vi "AddSystemIDtoCaliFile.vi"() -> ()   [LabVIEW 2020]
panel:
  out "error out":errorcluster
  in  "SYstemID":string(combo)="UCDMC"
  in  "error in (no error)":errorcluster
  out "selected path":path
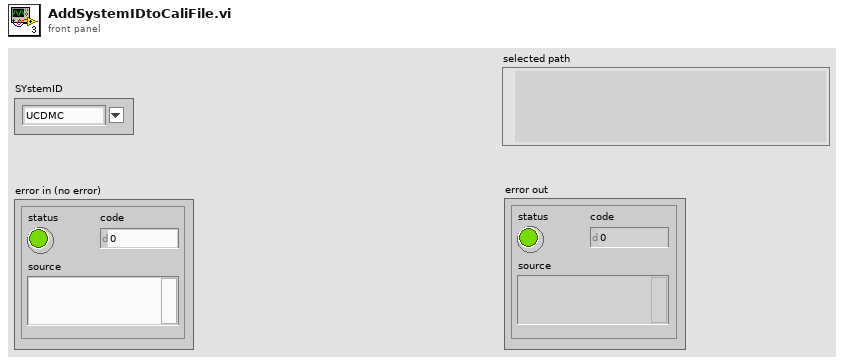
[diagram p1: front panel]
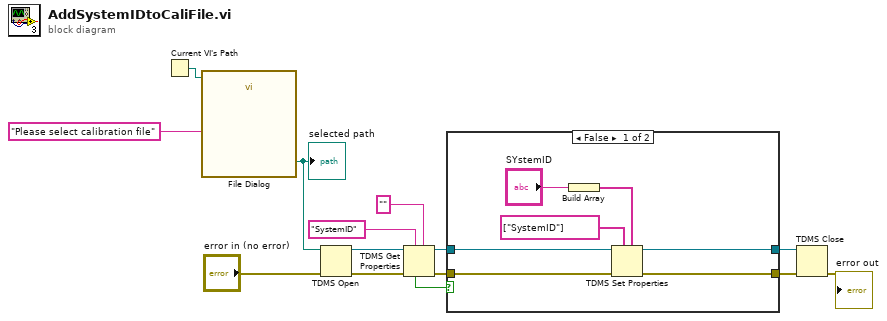
[diagram p0: block diagram]
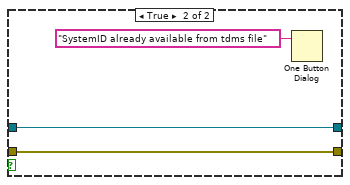
[diagram p2: hidden frame]
diagram:
  n1 = Current VI's Path() -> (path=w14:path)
  n2 = call "File Dialog"("start path"=w14, "prompt"="Please select calibration file") -> ("selected path"=w12:path)  [unwired: 10 in, 3 out]
  "selected path" <- w12
  n3 = TDMS Open(8:"error in (no error)", 11:w12) -> (0:w10:errorcluster, 3:w7:refnum<k34>)  [unwired: 5 in]
  n4 = TDMS Get Properties(5:"", 7:"SystemID" ("property name"), 8:w10, 11:w7) -> (0:w5:errorcluster, 3:w6:refnum<k34>, 6:w4:bool)  [unwired: 2 in, 3 out]
  n5 = case shown="False" w4 {
    tunnel: w6 -> [w18 w23]
    tunnel: w5 -> [w17 w22]
    tunnel: [w15 w23] -> w3
    tunnel: [w16 w22] -> w2
    frame False {
      n6 = Build Array("SYstemID") -> (w19:string[])
      n7 = TDMS Set Properties(5:w19, 7:string[] ["SystemID"] ("property names"), 8:w17, 11:w18) -> (0:w16:errorcluster, 3:w15:refnum<k34>)  [unwired: 2 in, 2 out]
    }
    frame True {
      n8 = One Button Dialog(message="SystemID already available from tdms file") -> ()  [unwired: 1 in, 1 out]
    }
  }
  n9 = TDMS Close(8:w2, 11:w3) -> (0:→"error out":errorcluster)  [unwired: 1 out]
